vi "portInit.vi"() -> ()   [LabVIEW 2018]
uses:
  <vilib>/Instr/_visa.llb/VISA Configure Serial Port (Instr).vi
panel:
  out "Combo Box":string(combo)
  out "位置":string
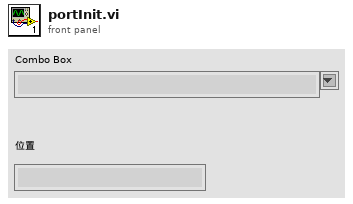
[diagram p1: front panel]
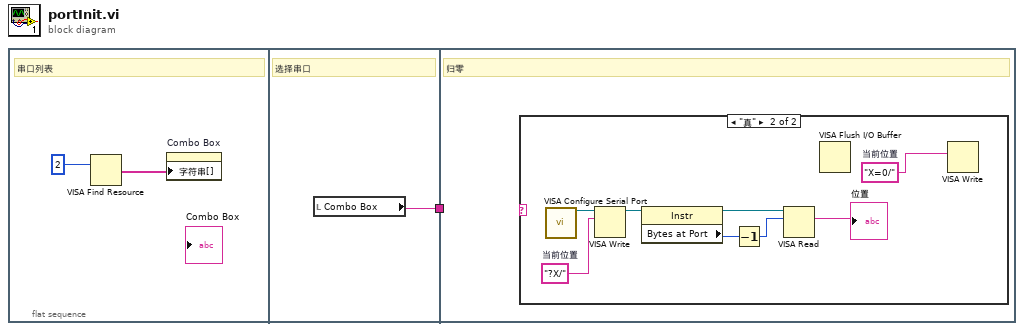
[diagram p0: block diagram]
diagram:
  n1 = flat-sequence {
    tunnel: [w4] -> w1
    tunnel: w1 -> [_]
    frame #0 {
      # "串口列表"
      n2 = VISA Find Resource(10:2) -> (3:w3:string[])  [unwired: 2 in, 2 out]
      n3 = property on="Combo Box" class="CmbBox"("字符串[]"=w3) -> ()  [unwired: 2 in, 2 out]
    }
    frame #1 {
      # "选择串口"
      n4 = local read "Combo Box"() -> (w4:string)
    }
    frame #2 {
      # "归零"
      n5 = case shown="\"真\"" {
        selector: _ -> [_ _]
        frame "假", Default {
        }
        frame "真" {
          w6 = "X=0/"  # 当前位置
          w5 = "?X/"  # 当前位置
          n6 = call-poly "VISA Configure Serial Port"() -> ("VISA resource name out"=w9:refnum<visa-resource-name>)  [unwired: 14 in, 1 out]
          n7 = VISA Write(VISA resource name=w9, write buffer=w5) -> (VISA resource name out=w10:refnum<visa-resource-name>)  [unwired: 1 in, 2 out]
          n8 = property class="Instr"(reference=w10) -> (reference out=w8:refnum<visa-resource-name>, "Bytes at Port"=w11:u32)  [unwired: 1 in, 1 out]
          n9 = Decrement(x=w11) -> (x-1=w12:u32)
          n10 = VISA Read(VISA resource name=w8, byte count=w12) -> (VISA resource name out=w13:refnum<visa-resource-name>, read buffer=→"位置":string)  [unwired: 1 in, 2 out]
          n11 = VISA Flush I/O Buffer() -> ()  [unwired: 3 in, 2 out]
          n12 = VISA Write(write buffer=w6) -> ()  [unwired: 2 in, 3 out]
        }
      }
    }
  }
